vi "主VI.vi"() -> ()   [LabVIEW 8.6]
panel:
  in  "簇":T1
  out "节气门\n开度电压":dbl(graph)
  out "档位":T2
  out "水温电压":dbl(graph)
  out "仪表控制项":T3 {"输出轴转速r/min" scale=0.0..5000.0; "发动机转速r/min" scale=0.0..5000.0; "车速km/h" scale=0.0..250.0}
  out "水温":dbl(knob) scale=0.0..120.0
  in  "节气门开度":dbl(knob) scale=0.0..100.0
  out "当前时间":timestamp format="%<当前时间%H时%M分%S秒>T"
  in  "关于...":bool
  in  "退出":bool
  # "汽车自动变速器运行监测系统"
  # "正常行驶用于显示汽车在正常行驶的时候各项参数变化，本模块可以实时显示汽车参数动态"
  # "本模块显示的是当汽车不受控制时，各项参数随节气门开度的变化情况。本模块可以时时显示汽车参数动态变化情况"
  # "本模块着重显示油压随节气门开度的变化情况，同时可以实时显示汽车各参数随节气门开度的变化情况"
  # "该部分作为备用模块作为今后系统的拓展与完善。目前尚未添加。"
  # "个人能力有限，毕业设计费尽千辛万苦，询问八方高人，但在坎坷与波折中受益匪浅，内含个人联系信息。"
  # "07汽服2班   某某某    基于labview的汽车自动变速器运行监测系统"
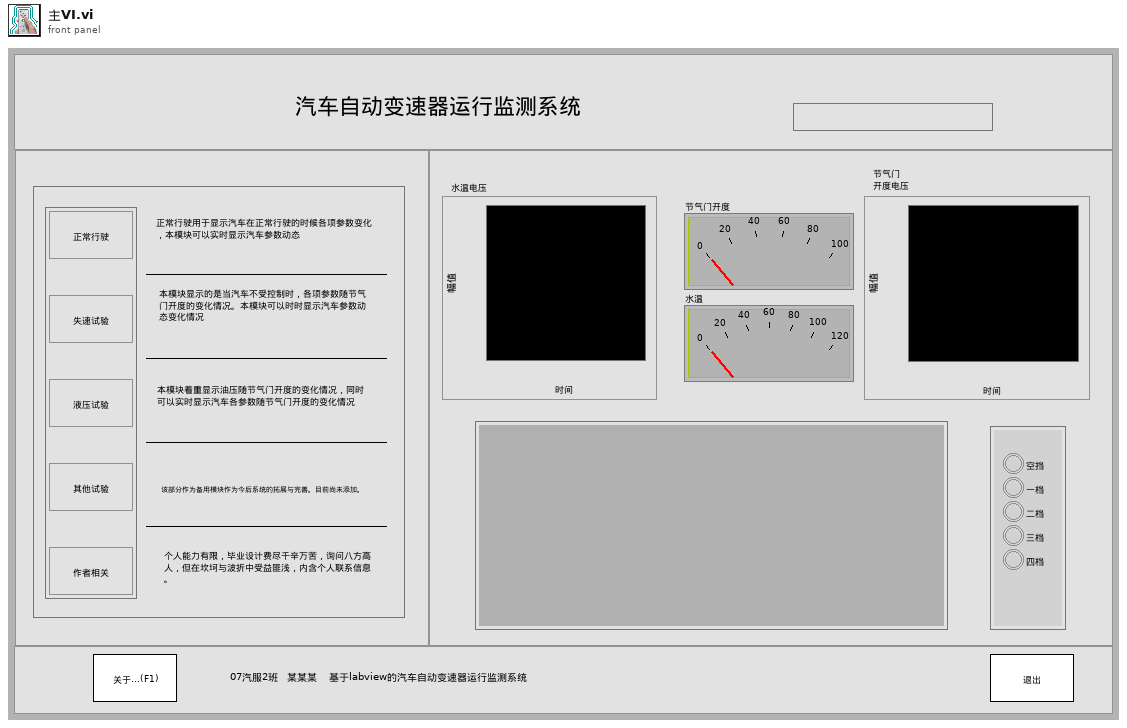
[diagram p1: front panel]
types:
  T1 = cluster{"正常行驶":bool, "失速试验":bool, "液压试验":bool, "文档核对":bool, "作者相关":bool}
  T2 = cluster{"空挡":bool, "一档":bool, "二档":bool, "三档":bool, "四档":bool}
  T3 = cluster{"车速km/h":dbl, "发动机转速r/min":dbl, "输出轴转速r/min":dbl, "报警灯":bool}
  T4 = cluster{"[0]":bool, "[1]":bool, "[2]":bool, "[3]":bool, "[4]":bool}
  T5 = cluster{"簇[0]":bool, "簇[1]":bool, "簇[2]":bool, "簇[3]":bool, "簇[4]":bool}
  T6 = cluster{"数组[0]":bool, "数组[1]":bool, "数组[2]":bool, "数组[3]":bool, "数组[4]":bool}
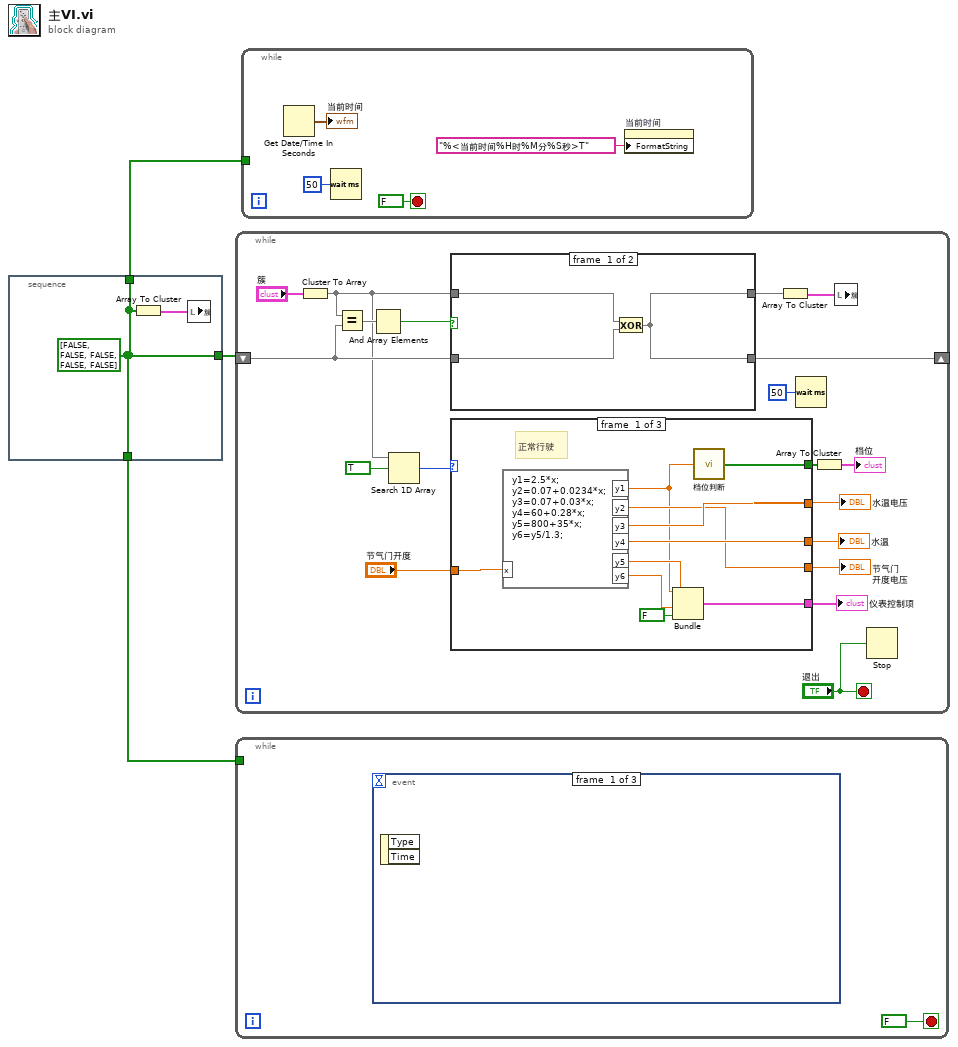
[diagram p0: block diagram]
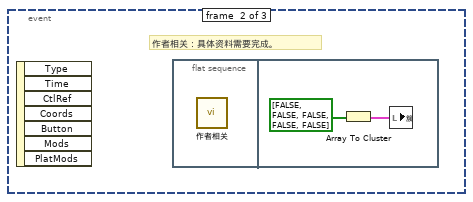
[diagram p2: hidden frame]
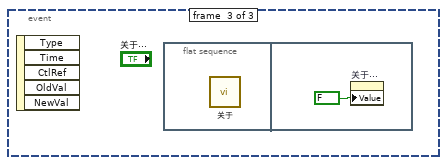
[diagram p3: hidden frame]
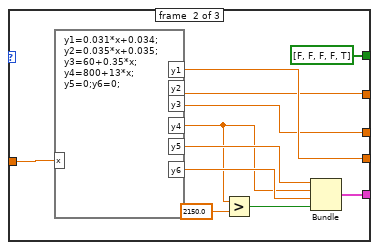
[diagram p5: hidden frame]
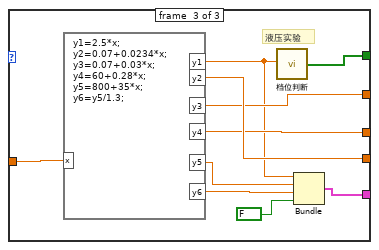
[diagram p6: hidden frame]
diagram:
  n1 = stacked-sequence {
    tunnel: [w4] -> w3
    tunnel: [w4] -> w2
    tunnel: [w4] -> w1
    frame #0 {
      w4 = bool[] [FALSE, FALSE, FALSE, FALSE, FALSE]
      n2 = Array To Cluster(array=w4) -> (cluster=w5:T4)
      n3 = local write "簇"(w5) -> ()
    }
  }
  n4 = while {
    shift-right: [w20] -> _
    shift-left: w3 -> [w21]
    stop <- "退出" stop-if-true
    n5 = Cluster To Array(cluster="簇") -> (array=w16:bool[])
    n6 = Equal?(x=w16, y=w21) -> (x = y?=w23:bool[])
    n7 = And Array Elements(Boolean array=w23) -> (logical AND=w22:bool)
    n8 = Search 1D Array(1D array=w16, element=TRUE ("元素")) -> (index of element=w6:i32)  [unwired: 1 in]
    n9 = case shown="真" w22 {
      tunnel: w16 -> [w27 w29]
      tunnel: w21 -> [w26 w28]
      tunnel: [w25 w28] -> w20
      tunnel: [w25 w29] -> w19
      frame #0 {
        n10 = Exclusive Or(1:w26, 2:w27) -> (0:w25:bool[])
      }
      frame #1 {
      }
    }
    n11 = case shown="1" w6 {
      tunnel: "节气门开度" -> [w39 w50 w60]
      tunnel: [w35 w42 w56] -> w13
      tunnel: [w34 w48 w54] -> w12
      tunnel: [w33 w40 w53] -> w11
      tunnel: [w32 w49 w55] -> w10
      tunnel: [w31 bool[] [FALSE, FALSE, FALSE, FALSE, TRUE] w52] -> w8
      frame #0 {
        # "正常行驶"
        n12 = formula code="y1=2.5*x;\ny2=0.07+0.0234*x;\ny3=0.07+0.03*x;\ny4=60+0.28*x;\ny5=800+35*x;\ny6=y5/1.3;"("x"=w39) -> ("y1"=w30:dbl, "y2"=w32:dbl, "y3"=w33:dbl, "y4"=w34:dbl, "y5"=w38:dbl, "y6"=w37:dbl)
        n13 = Bundle("y1"=w30, "y5"=w38, "y6"=w37, FALSE) -> (w35:cluster{"y1":dbl, "y5":dbl, "y6":dbl, bool})  [unwired: 1 in]
        n14 = call "档位判断.vi"("数值"=w30) -> ("数组"=w31:bool[])
      }
      frame #1 {
        # "失速行驶"
        n15 = formula code="y1=0.031*x+0.034;\ny2=0.035*x+0.035;\ny3=60+0.35*x;\ny4=800+13*x;\ny5=0;y6=0;"("x"=w50) -> ("y1"=w49:dbl, "y2"=w40:dbl, "y3"=w48:dbl, "y4"=w45:dbl, "y5"=w47:dbl, "y6"=w46:dbl)
        n16 = Greater?(x=w45, y=2150.0) -> (0:w43:bool)
        n17 = Bundle("y5"=w47, "y4"=w45, "y6"=w46, w43) -> (w42:cluster{"y5":dbl, "y4":dbl, "y6":dbl, bool})  [unwired: 1 in]
      }
      frame #2 {
        # "液压实验"
        n18 = formula code="y1=2.5*x;\ny2=0.07+0.0234*x;\ny3=0.07+0.03*x;\ny4=60+0.28*x;\ny5=800+35*x;\ny6=y5/1.3;"("x"=w60) -> ("y1"=w51:dbl, "y2"=w55:dbl, "y3"=w53:dbl, "y4"=w54:dbl, "y5"=w59:dbl, "y6"=w58:dbl)
        n19 = call "档位判断.vi"("数值"=w51) -> ("数组"=w52:bool[])
        n20 = Bundle("y1"=w51, "y5"=w59, "y6"=w58, FALSE) -> (w56:cluster{"y1":dbl, "y5":dbl, "y6":dbl, bool})  [unwired: 1 in]
      }
    }
    "水温" <- w12
    "仪表控制项" <- w13
    "水温电压" <- w11
    "节气门\n开度电压" <- w10
    n21 = Array To Cluster(array=w19) -> (cluster=w18:T5)
    n22 = Wait (ms)(milliseconds to wait=u32 50 ("等待时间（毫秒）")) -> ()  [unwired: 1 out]
    n23 = Array To Cluster(array=w8) -> (cluster=→"档位":T6)
    n24 = local write "簇"(w18) -> ()
    n25 = Stop(stop? (T)="退出") -> ()
  }
  n26 = while {
    tunnel: w1 -> [_]
    stop <- FALSE stop-if-true
    n27 = event shown="[1] \"簇.作者相关\": 鼠标按下" {
      selector: _ -> [_ _ _]
      dyn-events: _ -> [_ _ _]
      timeout: _ -> [_ _ _]
      event #0 {
        n28 = event-data() -> ()  [unwired: 1 in, 2 out]
      }
      event #1 {
        # "作者相关：具体资料需要完成。"
        n29 = event-data() -> ()  [unwired: 1 in, 7 out]
        n30 = flat-sequence {
          frame #0 {
            n31 = call "作者相关.vi"() -> ()  [unwired: 1 in]
          }
          frame #1 {
            n32 = Array To Cluster(array=bool[] [FALSE, FALSE, FALSE, FALSE, FALSE]) -> (cluster=w63:T4)
            n33 = local write "簇"(w63) -> ()
          }
        }
      }
      event #2 {
        n34 = event-data() -> ()  [unwired: 1 in, 5 out]
        n35 = flat-sequence {
          frame #0 {
            n36 = call "关于.vi"() -> ()  [unwired: 1 in]
          }
          frame #1 {
            n37 = property on="关于..." class="Bool (严格)"("Value"=FALSE ("关于...")) -> ()  [unwired: 2 in, 2 out]
          }
        }
      }
    }
  }
  n38 = while {
    tunnel: w2 -> [_]
    stop <- FALSE stop-if-true
    n39 = Get Date/Time In Seconds() -> (seconds since 1Jan1904=→"当前时间":timestamp)
    n40 = Wait (ms)(milliseconds to wait=u32 50 ("等待时间（毫秒）")) -> ()  [unwired: 1 out]
    n41 = property on="当前时间" class="AbsTime (严格)"("FormatString"="%<当前时间%H时%M分%S秒>T" ("格式字符串")) -> ()  [unwired: 2 in, 2 out]
  }
